vi "CRYView Pic Out Log.vi"(6 "vi reference":refnum<vi>, 11 "sData":string) -> ()   [LabVIEW 2013]
uses:
  SubVI/CRYMain Sub Window Global.vi
  CRYView Global.vi
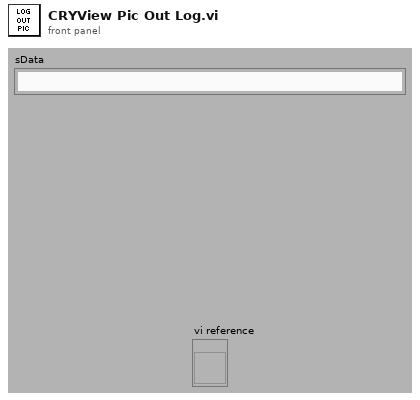
[diagram p1: front panel]
types:
  T1 = enum16{"open", "open or create", "create or replace", "create", "open (read only)"}
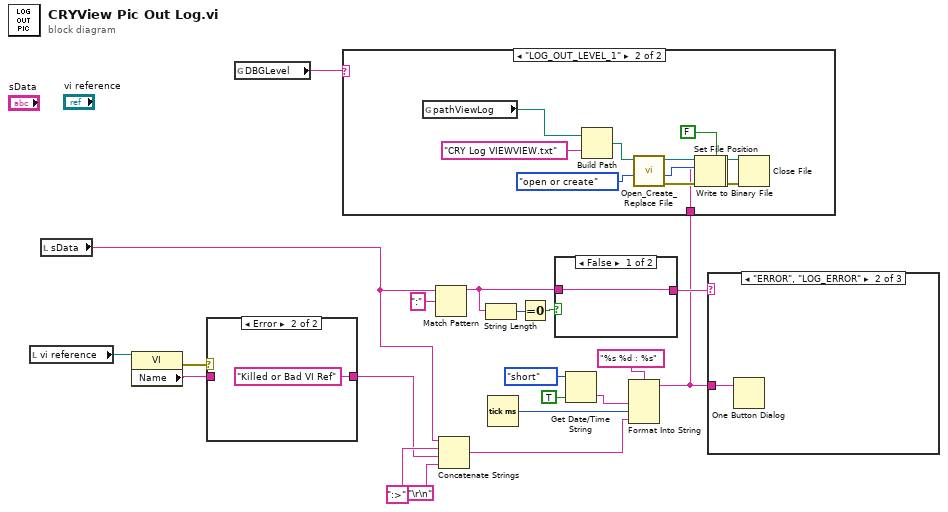
[diagram p0: block diagram]
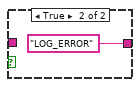
[diagram p4: hidden frame]
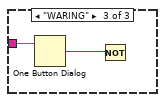
[diagram p6: hidden frame]
diagram:
  n1 = local read "vi reference"() -> (w20:refnum<vi>)
  n2 = local read "sData"() -> (w16:string)
  n3 = property class="VI"(reference=w20) -> (error out=w10:errorcluster, "Name"=w9:string)  [unwired: 1 in, 1 out]
  n4 = case shown="Error" w10 {
    tunnel: w9 -> [w21 _]
    tunnel: [w21 "Killed or Bad VI Ref" ("Name")] -> w15
    frame No Error {
    }
    frame Error {
    }
  }
  n5 = global read "CRYMain Sub Window Global.vi" "DBGLevel"() -> (w1:string)
  n6 = Match Pattern(string=w16, regular expression=":") -> (before substring=w12:string)  [unwired: 1 in, 3 out]
  n7 = Concatenate Strings(w16, ":>" ("string"), w15, "\r\n") -> (w3:string)
  n8 = String Length(string=w12) -> (length=w14:i32)
  n9 = Tick Count (ms)() -> (millisecond timer value=w4:u32)
  n10 = Equal To 0?(x=w14) -> (x = 0?=w13:bool)
  n11 = case shown="False" w13 {
    tunnel: [w23 "LOG_ERROR" ("sData")] -> w11
    tunnel: w12 -> [w23 _]
    frame False {
    }
    frame True {
    }
  }
  n12 = Get Date/Time String(date format (0)=enum16{"short", "long", "abbreviated"}."short", want seconds? (F)=TRUE) -> (time string=w5:string)  [unwired: 1 in, 1 out]
  n13 = Format Into String(format string="%s %d : %s", w5, w4, w3) -> (resulting string=w2:string)  [unwired: 2 in, 1 out]
  n14 = case shown="\"LOG_OUT_LEVEL_1\"" w1 {
    tunnel: w2 -> [_ w25]
    frame Default {
    }
    frame "LOG_OUT_LEVEL_1" {
      n15 = global read "CRYView Global.vi" "pathViewLog"() -> (w26:path)
      n16 = Build Path(base path=w26, name or relative path="CRY Log VIEWVIEW.txt" ("name")) -> (appended path=w27:path)
      n17 = call <vilib>:"Open_Create_Replace File.vi"("function (open:0)"=T1."open or create", "file path"=w27) -> ("error out"=w35:errorcluster, "file size (bytes)"=w33:i32, "refnum"=w34:refnum<file>)  [unwired: 6 in, 1 out]
      n18 = Set File Position(offset (in bytes) (0)=w33, refnum=w34, error in=w35) -> (refnum out=w30:refnum<file>, error out=w29:errorcluster)  [unwired: 1 in]
      n19 = Write to Binary File(file (use dialog)=w30, data=w25, error in=w29, 5:FALSE ("prepend array or string size? (T)")) -> (refnum out=w31:refnum<file>, error out=w32:errorcluster)  [unwired: 2 in, 1 out]
      n20 = Close File(refnum=w31, error in=w32) -> ()  [unwired: 2 out]
    }
  }
  n21 = case shown="\"ERROR\", \"LOG_ERROR\"" w11 {
    tunnel: w2 -> [_ w38 w39]
    frame Default {
    }
    frame "ERROR", "LOG_ERROR" {
      n22 = One Button Dialog(message=w38) -> ()  [unwired: 1 in, 1 out]
    }
    frame "WARING" {
      n23 = One Button Dialog(message=w39) -> (true=w40:bool)  [unwired: 1 in]
      n24 = Not(x=w40) -> ()  [unwired: 1 out]
    }
  }
